vi "IsEqual.vi"(2 "is equal to":refnum<class>, 3 "reference in":refnum<class "G#Interface.lvclass">) -> (0 "is equal?":bool, 1 "reference out":refnum<class "G#Interface.lvclass">)   [LabVIEW 2020, in "G#Interface.lvclass"]
doc: "Checks if the two input object references are one and the same object."
uses:
  G#Interface.lvclass
  G#Object/G#Object.lvclass
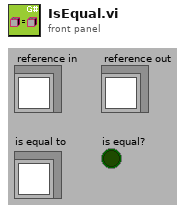
[diagram p1: front panel]
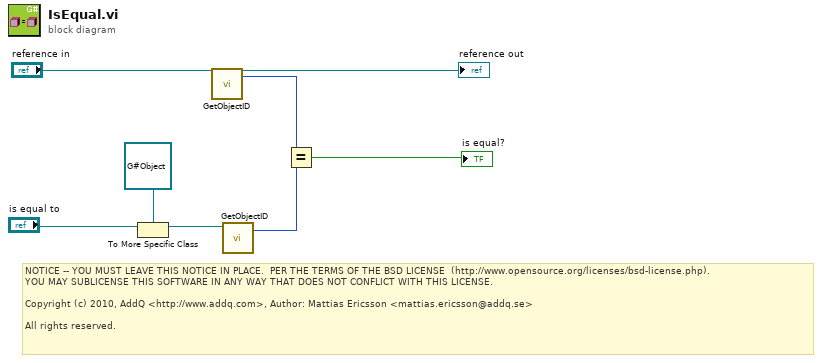
[diagram p0: block diagram]
diagram:
  # "NOTICE -- YOU MUST LEAVE THIS NOTICE IN PLACE.  PER THE TERMS OF THE BSD LICENSE  (http://www.opensource.org/licenses/bsd-license.php).\nYOU MAY SUBLICENSE THIS SOFTWARE IN ANY WAY THAT DOES NOT CONFLICT WITH THIS LICENSE.\n\nCopyright (c) 2010, AddQ <http://www.addq.com>, Author: Mattias Ericsson <mattias.ericsson@addq.se>\n\nAll rights reserved."
  n1 = To More Specific Class(target class=refnum<class "G#Object.lvclass"> refnum ("G#Object.lvclass"), reference="is equal to") -> (specific class reference=w2:refnum<class "G#Object.lvclass">)  [unwired: 1 in, 1 out]
  n2 = call-dynamic "GetObjectID.vi"("reference in"="reference in") -> ("reference out"=→"reference out":refnum<class "G#Interface.lvclass">, "object ID"=w7:u32)  [unwired: 16 in, 1 out]
  n3 = call-dynamic "GetObjectID.vi"("reference in"=w2) -> ("object ID"=w6:u32)  [unwired: 16 in, 2 out]
  n4 = Equal?(x=w7, y=w6) -> (x = y?=→"is equal?":bool)
